vi "New ADS1X15 Device.vi"(8 "error in (no error)":errorcluster, 10 "SPI CS Line":u8=72 format="%.0x", 11 "I2C":refnum<class "LINX SPI.lvclass">) -> (0 "error out":errorcluster, 3 "LINX-ADS1X15 out":refnum<class "LINX-ADS1256.lvclass">)   [LabVIEW 2020, in "LINX-ADS1256.lvclass"]
uses:
  LINX-ADS1256.lvclass
  LINX SPI/LINX SPI.lvclass
  <vilib>/MakerHub/LINX/Private/Type Defs/Peripherals/SPI/SPI CS Logic Level.ctl
  <vilib>/MakerHub/LINX/LMH-LINX.lvlib
  <vilib>/MakerHub/LINX/Public/Peripherals/SPI/SPI CS Config.ctl
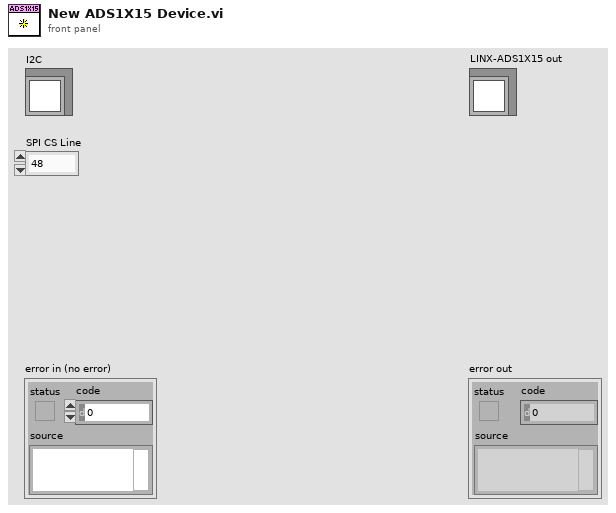
[diagram p1: front panel]
types:
  T1 = typedef "LMH-LINX.lvlib/SPI CS Config.ctl" = cluster{"CS Channel":u8, "CS Logic Level":T2}
  T2 = typedef "LMH-LINX.lvlib/SPI CS Logic Level.ctl" = enum8{"Active Low", "Active High"}
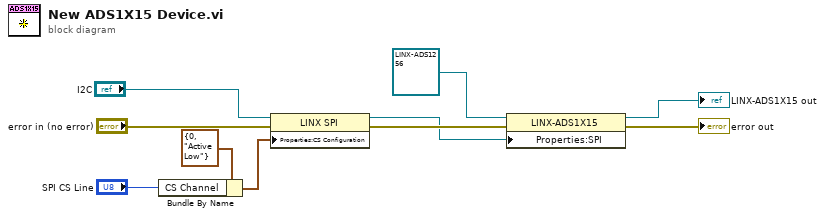
[diagram p0: block diagram]
diagram:
  n1 = Bundle By Name(cluster=T1 {"CS Channel"=0, "CS Logic Level"=enum."Active Low"} ("CS Configuration"), "CS Channel"="SPI CS Line") -> (w2:T1)
  n2 = property class="LINX SPI"(reference="I2C", error in="error in (no error)", "Properties:CS Configuration"=w2) -> (reference out=w7:refnum<class "LINX SPI.lvclass">, error out=w8:errorcluster)
  n3 = property class="LINX-ADS1X15"(reference=refnum<class "LINX-ADS1256.lvclass"> refnum ("LINX-ADS1X15 in"), error in=w8, "Properties:SPI"=w7) -> (reference out=→"LINX-ADS1X15 out":refnum<class "LINX-ADS1256.lvclass">, error out=→"error out":errorcluster)
